vi "Scott -- strain -- save sweep V0.vi"(7 "sweep folder name":path=path "D:/Technique/Strain/URu2Si2-xPx/x=0.01/141113 URu2Si2 0p01 eyy ryy.dat", 9 "data":dbl[][](array[numeric]), 10 "temperature":dbl=114.59, 11 "strain sweep control":T1={"just in case"=TRUE, "Piezo Amplifier settings"={"Gain "=69.44, "offset (V)"=69.44}, "voltage-parameters-IN"={"phase "=2.88, "amplitude (V)"=-0.7854, "offset (V)"=0.28, "time delay (sec)"=0.5, "period (sec)"=50.0, "shape"=enum."triangle"}, "Lockin Settings"=[{"Offset"=FALSE, "GPIB Address"=6}, {"Offset"=TRUE, "GPIB Address"=7}], "VISA address Agilent  IN"="", "number of iterations"=1.0, "Piezo sweep settings"={"max Piezo voltage (V) "=69.44, "min Piezo voltage (V)"=69.44, "delay (sec)"=69.44, "period (sec)"=69.44, "shape"=enum."triangle"}}) -> ()   [LabVIEW 2014]
uses:
  Scott -- strain -- strain sweep control.ctl
  FSU/ScottRiggs/Piezo2/voltage-wave-generator-parameters.ctl
  file -- scan filename action.ctl
  file -- read-write control.ctl
  <vilib>/Utility/libraryn.llb/Check if File or Folder Exists.vi
  <vilib>/Utility/file.llb/Write To Spreadsheet File (DBL).vi
panel:
  out "concatenated string":string
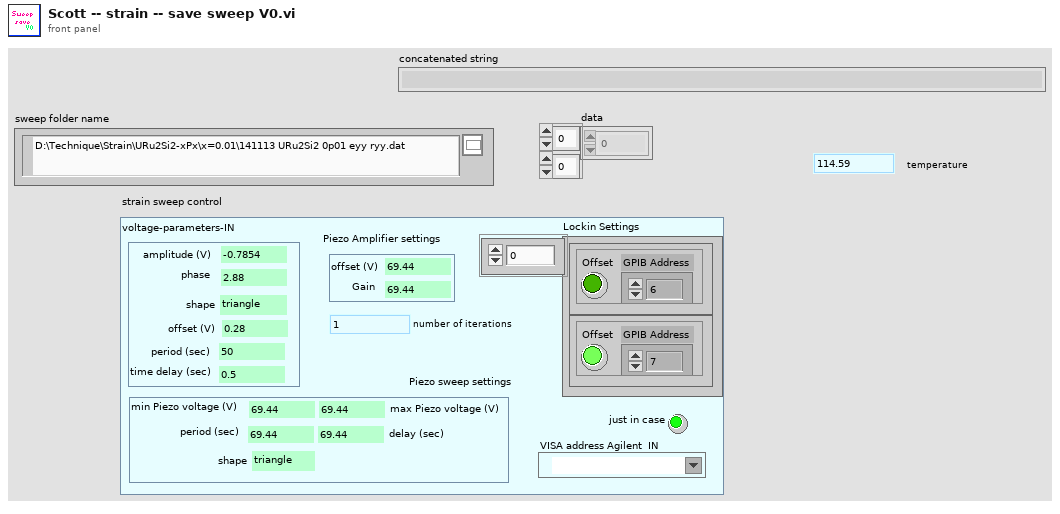
[diagram p1: front panel]
types:
  T1 = typedef "Scott -- strain -- strain sweep control.ctl" = cluster{"just in case":bool, "Piezo Amplifier settings":cluster{"Gain ":dbl, "offset (V)":dbl}, "voltage-parameters-IN":T2, "Lockin Settings":cluster{"Offset":bool, "GPIB Address":i16}[], "VISA address Agilent  IN":refnum<visa-resource-name>, "number of iterations":dbl, "Piezo sweep settings":cluster{"max Piezo voltage (V) ":dbl, "min Piezo voltage (V)":dbl, "delay (sec)":dbl, "period (sec)":dbl, "shape":enum16{"triangle", "sine", "none"}}}
  T2 = typedef "voltage-wave-generator-parameters.ctl" = cluster{"phase ":dbl, "amplitude (V)":dbl, "offset (V)":dbl, "time delay (sec)":dbl, "period (sec)":dbl, "shape":enum16{"triangle", "sine", "none"}}
  T3 = typedef "file -- read-write control.ctl" = enum16{"read", "write all", "append one line"}
  T4 = typedef "file -- scan filename action.ctl" = enum16{"prefix base name", "datestring regexp", "parse datestring", "datestring", "filename regexp", "parse filename", "datestring regexp (no brackets)", "suffix base name"}
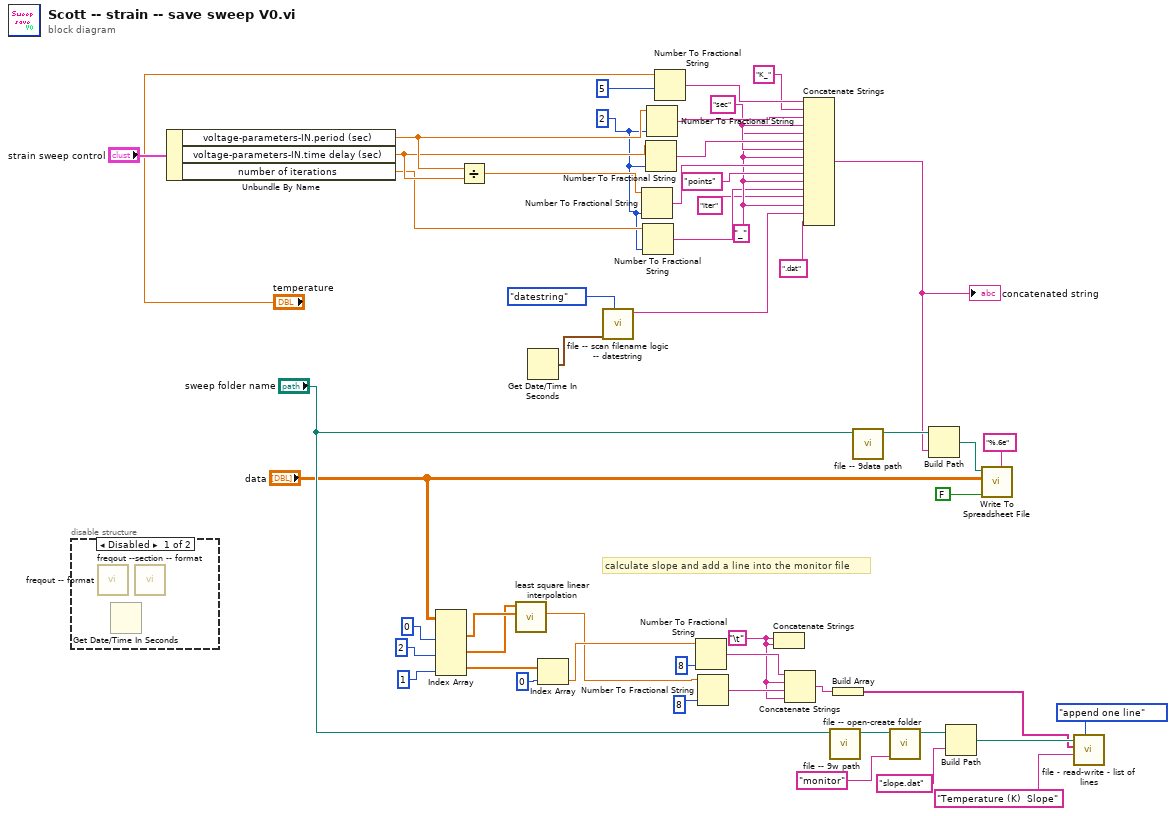
[diagram p0: block diagram]
diagram:
  w8 = "\t"
  w26 = i16 2 ("width (-)")
  w41 = "sec" ("string")
  w33 = "_" ("string")
  # "calculate slope and add a line into the monitor file"
  n1 = disable-structure shown="Disabled" {
    frame Disabled {
      n2 = call "freqout -- format.vi"() -> ()  [unwired: 11 in, 1 out]
      n3 = Get Date/Time In Seconds() -> ()  [unwired: 1 out]
      n4 = call "freqout --section -- format.vi"() -> ()  [unwired: 11 in, 1 out]
    }
    frame Enabled {
    }
  }
  n5 = Unbundle By Name("strain sweep control") -> ("voltage-parameters-IN.period (sec)"=w40:dbl, "voltage-parameters-IN.time delay (sec)"=w39:dbl, "number of iterations"=w37:dbl)
  n6 = Index Array(array="data", index (col) #1=0 ("index"), index (col) #2=2 ("index"), index (col) #3=1 ("index")) -> (element #1=w2:dbl[], element #2=w1:dbl[], element #3=w13:dbl[])  [unwired: 3 in]
  n7 = Divide(x=w40, y=w39) -> (x/y=w38:dbl)
  n8 = call "least square linear interpolation.vi"("X"=w2, "Y"=w1) -> ("slope"=w5:dbl)  [unwired: 8 in, 1 out]
  n9 = Get Date/Time In Seconds() -> (seconds since 1Jan1904=w44:timestamp)
  n10 = Index Array(array=w13, index=0) -> (element=w6:dbl)
  n11 = call "file -- scan filename logic -- datestring.vi"("scan filename action"=file_--_scan_filename_action."datestring", "time stamp IN"=w44) -> ("date/time string OUT"=w47:string)  [unwired: 6 in, 3 out]
  n12 = Number To Fractional String(number=w38, precision (6)=w26) -> (F-format string=w35:string)  [unwired: 2 in]
  n13 = Number To Fractional String(number=w37, precision (6)=w26) -> (F-format string=w32:string)  [unwired: 2 in]
  n14 = Number To Fractional String(number=w39, precision (6)=w26) -> (F-format string=w42:string)  [unwired: 2 in]
  n15 = Number To Fractional String(number=w40, precision (6)=w26) -> (F-format string=w43:string)  [unwired: 2 in]
  n16 = Number To Fractional String(number="temperature", precision (6)=i16 5 ("width (-)")) -> (F-format string=w49:string)  [unwired: 2 in]
  n17 = Number To Fractional String(number=w6, precision (6)=i16 8) -> (F-format string=w11:string)  [unwired: 2 in]
  n18 = Number To Fractional String(number=w5, precision (6)=i16 8) -> (F-format string=w10:string)  [unwired: 2 in]
  n19 = Concatenate Strings(w8, w8) -> ()  [unwired: 1 out]
  n20 = Concatenate Strings(w11, w8, w10, w8) -> (w4:string)
  n21 = Concatenate Strings(w49, "K_" ("string"), w43, w41, w33, w42, w41, w33, w35, "points" ("string"), w33, w32, "iter" ("string"), w33, w47, ".dat" ("string")) -> (w28:string)
  "concatenated string" <- w28
  n22 = call "file -- 9w path.vi"("sweep folder"="sweep folder name") -> ("9w path"=w23:path)  [unwired: 10 in]
  n23 = Build Array(w4) -> (w3:string[])
  n24 = call "file -- 9data path.vi"("sweep folder"="sweep folder name") -> ("9data path"=w29:path)  [unwired: 10 in]
  n25 = call "file -- open-create folder.vi"("folder name"="monitor" ("name or relative path"), "base path"=w23) -> ("folder path out"=w22:path)  [unwired: 9 in]
  n26 = Build Path(base path=w29, name or relative path=w28) -> (appended path=w27:path)
  n27 = Build Path(base path=w22, name or relative path="slope.dat") -> (appended path=w20:path)
  n28 = call-poly <vilib>:"Write To Spreadsheet File.vi"("format (%.3f)"="%.6e", "append to file? (new file:F)"=FALSE, "2D data"="data", "file path (dialog if empty)"=w27) -> ()  [unwired: 4 in, 1 out]
  n29 = call "file - read-write - list of lines.vi"("read/write control"=file_--_read-write_control."append one line", "header"="Temperature (K)  Slope", "list of lines IN"=w3, "file path"=w20) -> ()  [unwired: 6 in, 2 out]
